vi "LimelightSeekerBasic.vi"() -> ()   [LabVIEW 2018]
uses:
  <vilib>/Rock Robotics/Network Tables/NT Read Number.vi
panel:
  in  "RotError":dbl
  in  "FinalForwardMS":u32
  out "Ts":dbl
  out "PrevFOV":bool
  out "Ta":dbl
  out "error out":errorcluster
  out "RightOut":dbl
  out "LeftOut":dbl
  in  "BaseSpeed":dbl=0.3
  out "Distance":dbl
  out "Deadband":bool
  out "RightFOV":bool
  out "LeftFOV":bool
  in  "AimMin":dbl
  in  "Camera angle":dbl=14.5
  in  "Camera height":dbl=0.3
  in  "Target height":dbl=1.4
  in  "kPDrive":dbl=1.0
  in  "kPAim":dbl=0.01
  in  "Translation Deadband":dbl=1.2
  in  "Target Area":dbl=16.0
  # "<-- This guy is a percentage of the image in decimal format. He can't go over 1.0 or below 0.0"
  # "<-- This guy is the \"acceptable\" translational error"
  # "<-- Proportionality constants"
  # "<-- Height of your target. This VARIES w cargo ship and rocket so we need a selector (thats a TODO)"
  # "<-- Height of camera from the ground"
  # "<-- Angle Camera makes from horizontal"
  # "<-- Minimum speed to adjust steering by, to avoid overshoot"
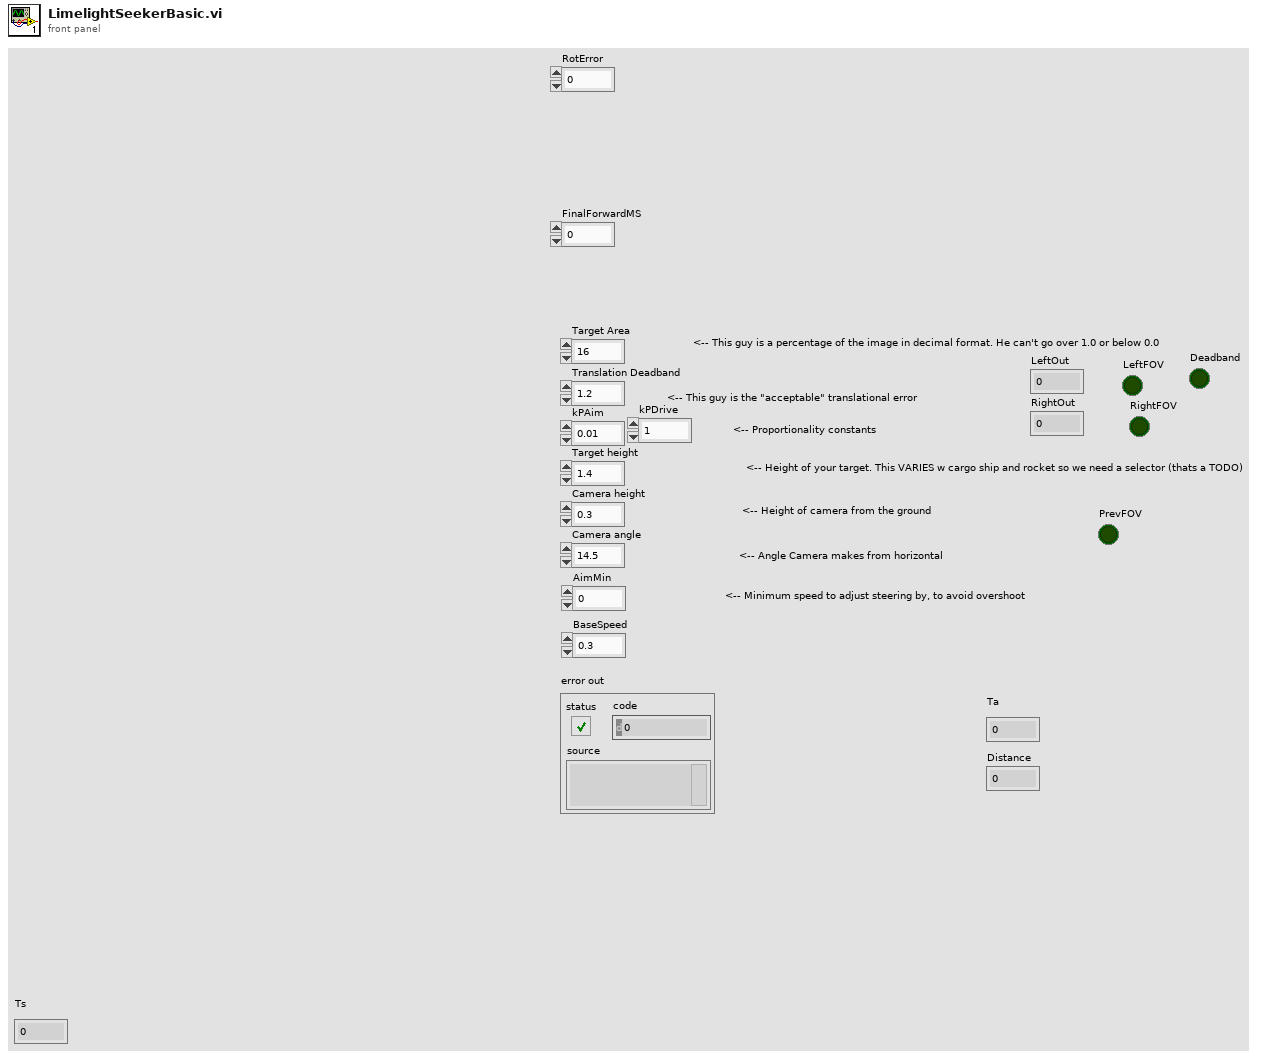
[diagram p1: front panel]
types:
  T1 = typedef "WPI_MotorControlDeviceRef.ctl" = cluster{"DeviceStatus":errorcluster, "Type":T2, "PWM":cluster{"PWM Channel":T3, "DeadBand":T4}, "CAN":cluster{"Device Number":u8, "SetOutput VI Ref":variant, "GetOutput VI Ref":variant, "Enable VI Ref":variant, "Disable VI Ref":variant, "Data":variant}, "Invert":bool, "DIO PWM":cluster{"PWM \"Enable\" Channel":T3, "DIOChannel":T5, "PWM Rate":dbl}}
  T2 = typedef "WPI_MotorControlType.ctl" = enum16{"PWM", "CAN", "DIO PWM"}
  T3 = typedef "FPGA_DIOPWMChannel.ctl" = enum8{"PWM 0", "PWM 1", "PWM 2", "PWM 3", "PWM 4", "PWM 5", "PWM 6", "PWM 7", "PWM 8", "PWM 9", "PWM MXP 0", "PWM MXP 1", "PWM MXP 2", "PWM MXP 3", "PWM MXP 4", "PWM MXP 5", "PWM MXP 6", "PWM MXP 7", "PWM MXP 8", "PWM MXP 9", "Invalid"}
  T4 = typedef "WPI_PWMDeadband.ctl" = cluster{"Name":string, "maxPositivePwm":i32, "minPositivePwm":i32, "centerPwm":i32, "maxNegativePwm":i32, "minNegativePwm":i32, "angularRange":u16}
  T5 = typedef "FPGA_DIOChannel.ctl" = enum8{"DIO 0", "DIO 1", "DIO 2", "DIO 3", "DIO 4", "DIO 5", "DIO 6", "DIO 7", "DIO 8", "DIO 9", "DIO MXP 0", "DIO MXP 1", "DIO MXP 2", "DIO MXP 3", "DIO MXP 4", "DIO MXP 5", "DIO MXP 6", "DIO MXP 7", "DIO MXP 8", "DIO MXP 9", "DIO MXP 10", "DIO MXP 11", "DIO MXP 12", "DIO MXP 13", "DIO MXP 14", "DIO MXP 15", "SPI Port CS1", "SPI Port CS2", "SPI Port CS3", "SPI Port MISO", "SPI Port MOSI", "Invalid"}
  T6 = cluster{"MotorControlDevRef":T1, "MotorControlDevRef":T1}
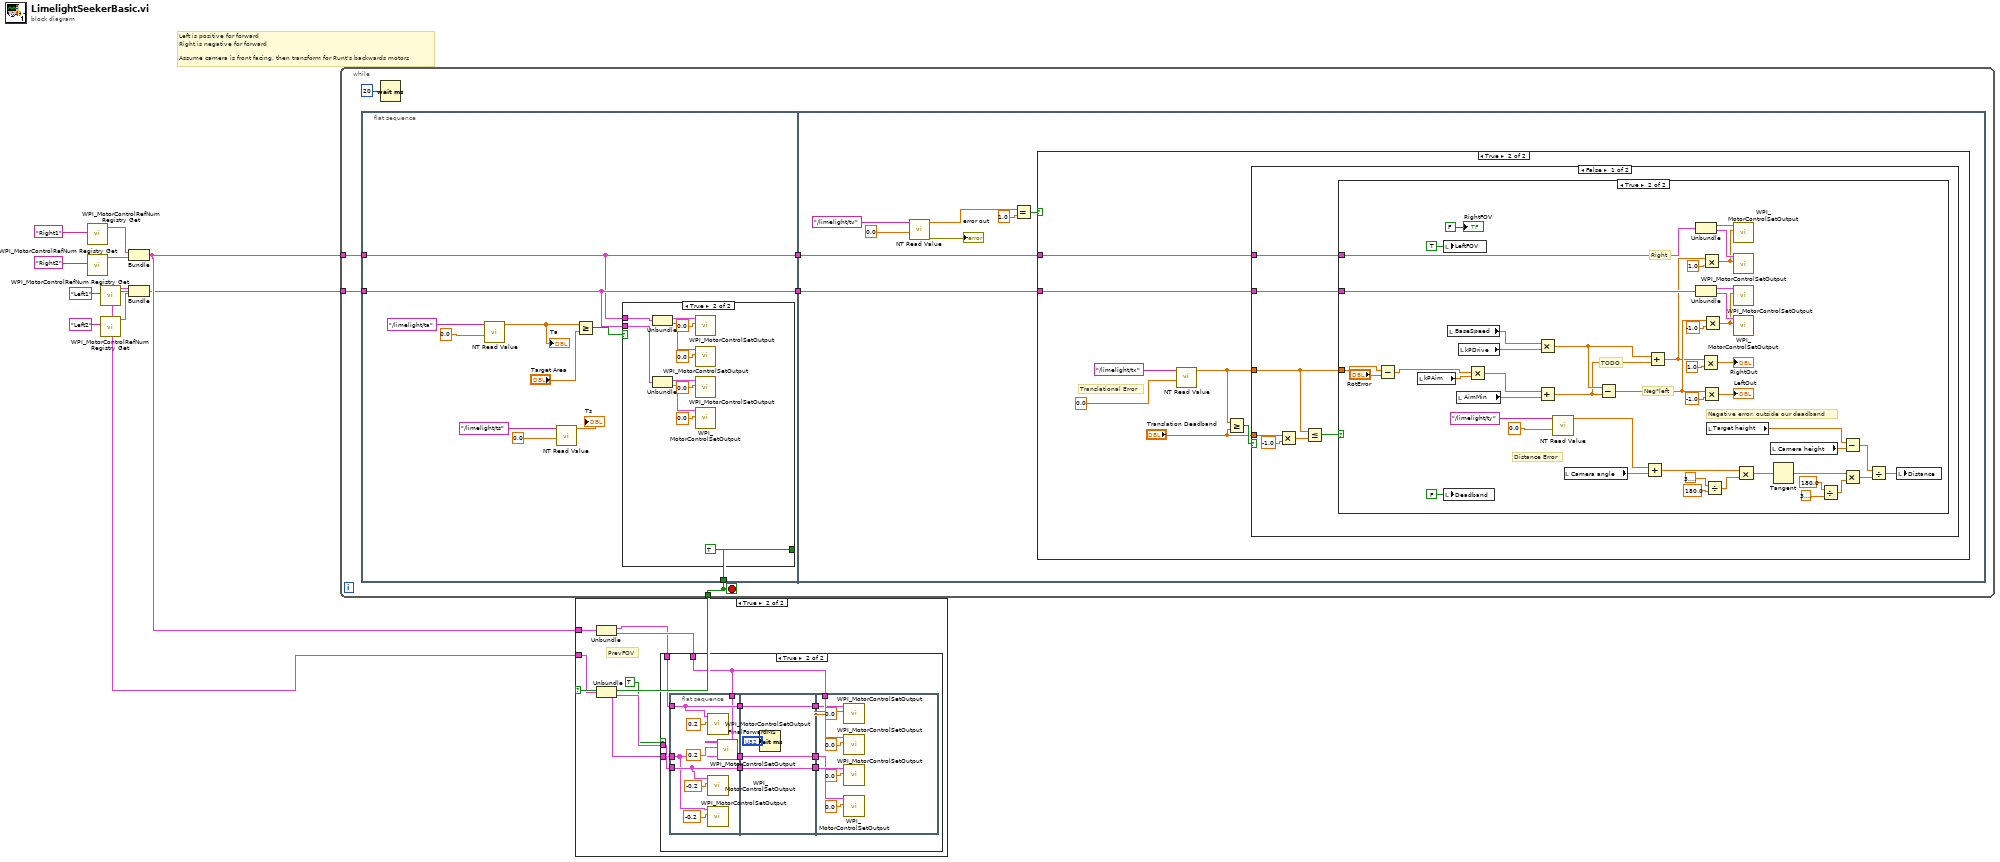
[diagram p0: block diagram]
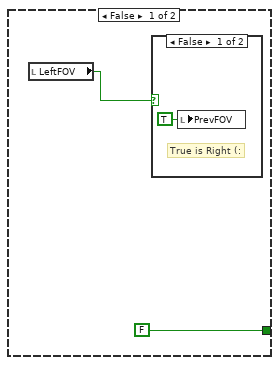
[diagram p4: hidden frame]
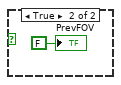
[diagram p5: hidden frame]
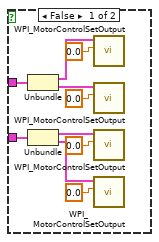
[diagram p6: hidden frame]
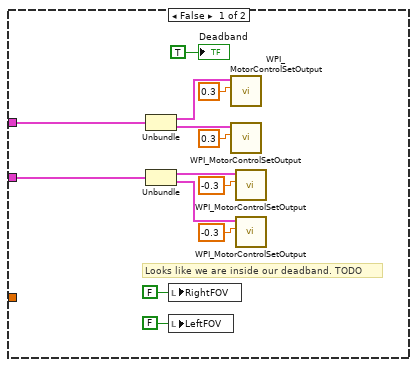
[diagram p7: hidden frame]
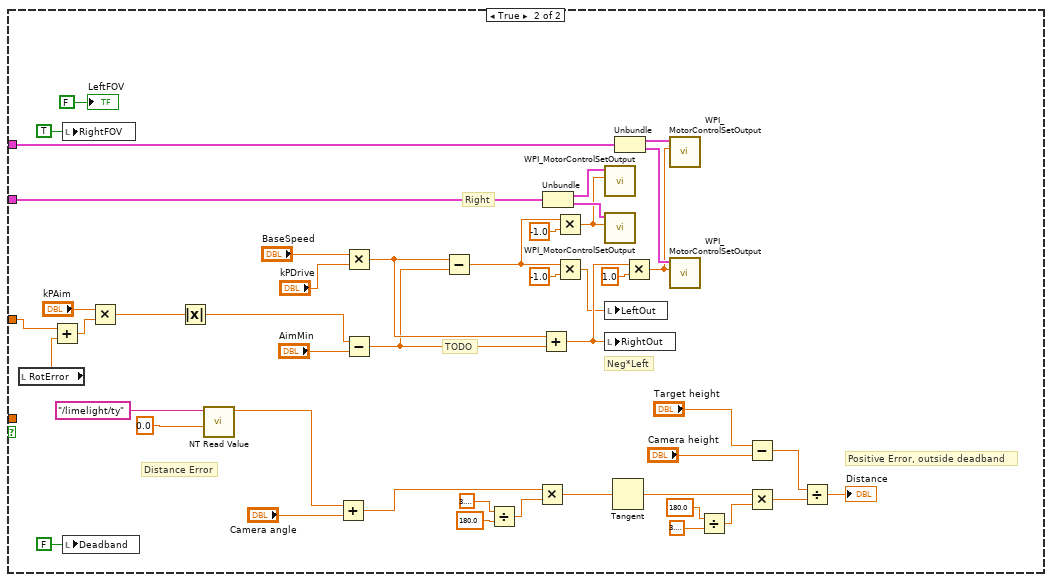
[diagram p8: hidden frame]
diagram:
  # "Left is positive for forward\nRight is negative for forward\n\nAssume camera is front facing, then transform for Runt's backwards motors"
  n1 = call <vilib>:"WPI_MotorControlRefNum Registry Get.vi"("refnum name"="Right1") -> ("MotorControlDevRef"=w5:T1)  [unwired: 9 in, 1 out]
  n2 = call <vilib>:"WPI_MotorControlRefNum Registry Get.vi"("refnum name"="Right2") -> ("MotorControlDevRef"=w4:T1)  [unwired: 9 in, 1 out]
  n3 = call <vilib>:"WPI_MotorControlRefNum Registry Get.vi"("refnum name"="Left1") -> ("MotorControlDevRef"=w7:T1)  [unwired: 9 in, 1 out]
  n4 = call <vilib>:"WPI_MotorControlRefNum Registry Get.vi"("refnum name"="Left2") -> ("MotorControlDevRef"=w6:T1)  [unwired: 9 in, 1 out]
  n5 = Bundle("MotorControlDevRef"=w5, "MotorControlDevRef"=w4) -> (w2:T6)  [unwired: 1 in]
  n6 = Bundle("MotorControlDevRef"=w7, "MotorControlDevRef"=w6) -> (w1:T6)  [unwired: 1 in]
  n7 = while {
    tunnel: w1 -> [w17]
    tunnel: w2 -> [w16]
    tunnel: [w12] -> w3
    stop <- w12 stop-if-true
    n8 = flat-sequence {
      tunnel: w16 -> [w24]
      tunnel: w17 -> [w25]
      tunnel: [w25] -> w15
      tunnel: [w24] -> w14
      tunnel: [w21] -> w12
      tunnel: w15 -> [w51]
      tunnel: w14 -> [w50]
      frame #0 {
        n9 = call-poly <vilib>:"NT Read Value.vi"("Default Value"=0.0, "Name"="/limelight/ta") -> ("Numeric"=w26:dbl)  [unwired: 8 in, 1 out]
        "Ta" <- w26
        n10 = call-poly <vilib>:"NT Read Value.vi"("Default Value"=0.0, "Name"="/limelight/ts") -> ("Numeric"=→"Ts":dbl)  [unwired: 8 in, 1 out]
        n11 = Greater Or Equal?(x=w26, y="Target Area") -> (x >= y?=w28:bool)
        n12 = case shown="True" w28 {
          tunnel: w25 -> [_ w43]
          tunnel: w24 -> [_ w42]
          tunnel: [FALSE TRUE] -> w21
          frame False {
            n13 = local read "LeftFOV"() -> (w29:bool)
            n14 = case shown="False" w29 {
              frame False {
                # "True is Right (:"
                n15 = local write "PrevFOV"(TRUE ("PrevFOV")) -> ()
              }
              frame True {
                "PrevFOV" <- FALSE ("PrevFOV")
              }
            }
          }
          frame True {
            n16 = Unbundle(w42) -> ("MotorControlDevRef"=w37:T1, "MotorControlDevRef"=w36:T1)
            n17 = Unbundle(w43) -> ("MotorControlDevRef"=w35:T1, "MotorControlDevRef"=w34:T1)
            n18 = call <vilib>:"WPI_MotorControlSetOutput.vi"("Output"=0.0, "MotorControlDevRef"=w37) -> ()  [unwired: 7 in, 3 out]
            n19 = call <vilib>:"WPI_MotorControlSetOutput.vi"("Output"=0.0, "MotorControlDevRef"=w36) -> ()  [unwired: 7 in, 3 out]
            n20 = call <vilib>:"WPI_MotorControlSetOutput.vi"("Output"=0.0, "MotorControlDevRef"=w35) -> ()  [unwired: 7 in, 3 out]
            n21 = call <vilib>:"WPI_MotorControlSetOutput.vi"("Output"=0.0, "MotorControlDevRef"=w34) -> ()  [unwired: 7 in, 3 out]
          }
        }
      }
      frame #1 {
        n22 = call-poly <vilib>:"NT Read Value.vi"("Default Value"=0.0, "Name"="/limelight/tv") -> ("error out"=→"error out":errorcluster, "Numeric"=w47:dbl)  [unwired: 8 in]
        n23 = Equal?(x=w47, y=1.0) -> (x = y?=w48:bool)
        n24 = case shown="True" w48 {
          tunnel: w51 -> [w52 w63]
          tunnel: w50 -> [w53 w62]
          frame False {
            n25 = Unbundle(w53) -> ("MotorControlDevRef"=w55:T1, "MotorControlDevRef"=w54:T1)
            n26 = Unbundle(w52) -> ("MotorControlDevRef"=w57:T1, "MotorControlDevRef"=w56:T1)
            n27 = call <vilib>:"WPI_MotorControlSetOutput.vi"("Output"=0.0, "MotorControlDevRef"=w55) -> ()  [unwired: 7 in, 3 out]
            n28 = call <vilib>:"WPI_MotorControlSetOutput.vi"("Output"=0.0, "MotorControlDevRef"=w54) -> ()  [unwired: 7 in, 3 out]
            n29 = call <vilib>:"WPI_MotorControlSetOutput.vi"("Output"=0.0, "MotorControlDevRef"=w57) -> ()  [unwired: 7 in, 3 out]
            n30 = call <vilib>:"WPI_MotorControlSetOutput.vi"("Output"=0.0, "MotorControlDevRef"=w56) -> ()  [unwired: 7 in, 3 out]
          }
          frame True {
            # "Translational Error"
            n31 = call-poly <vilib>:"NT Read Value.vi"("Default Value"=0.0, "Name"="/limelight/tx") -> ("Numeric"=w65:dbl)  [unwired: 8 in, 1 out]
            n32 = Greater Or Equal?(x=w65, y="Translation Deadband") -> (x >= y?=w66:bool)
            n33 = case shown="False" w66 {
              tunnel: w65 -> [w71 w137]
              tunnel: "Translation Deadband" -> [w73 _]
              tunnel: w63 -> [w70 w154]
              tunnel: w62 -> [w69 w153]
              frame False {
                n34 = Multiply(x=w73, y=-1.0) -> (x*y=w74:dbl)
                n35 = Less Or Equal?(x=w71, y=w74) -> (x <= y?=w72:bool)
                n36 = case shown="True" w72 {
                  tunnel: w71 -> [_ w90]
                  tunnel: w70 -> [w76 w107]
                  tunnel: w69 -> [w77 w106]
                  frame False {
                    # "Looks like we are inside our deadband. TODO"
                    n37 = Unbundle(w77) -> ("MotorControlDevRef"=w79:T1, "MotorControlDevRef"=w78:T1)
                    n38 = Unbundle(w76) -> ("MotorControlDevRef"=w81:T1, "MotorControlDevRef"=w80:T1)
                    n39 = local write "RightFOV"(FALSE ("RightFOV")) -> ()
                    n40 = local write "LeftFOV"(FALSE ("LeftFOV")) -> ()
                    n41 = call <vilib>:"WPI_MotorControlSetOutput.vi"("Output"=0.3, "MotorControlDevRef"=w79) -> ()  [unwired: 7 in, 3 out]
                    n42 = call <vilib>:"WPI_MotorControlSetOutput.vi"("Output"=0.3, "MotorControlDevRef"=w78) -> ()  [unwired: 7 in, 3 out]
                    n43 = call <vilib>:"WPI_MotorControlSetOutput.vi"("Output"=-0.3, "MotorControlDevRef"=w81) -> ()  [unwired: 7 in, 3 out]
                    n44 = call <vilib>:"WPI_MotorControlSetOutput.vi"("Output"=-0.3, "MotorControlDevRef"=w80) -> ()  [unwired: 7 in, 3 out]
                    "Deadband" <- TRUE ("Deadband")
                  }
                  frame True {
                    # "Right"
                    # "Neg*left"
                    # "TODO"
                    # "Distance Error"
                    # "Negative error, outside our deadband"
                    n45 = Subtract(x=w90, y="RotError") -> (x-y=w89:dbl)
                    n46 = local read "kPAim"() -> (w124:dbl)
                    n47 = local write "LeftFOV"(TRUE ("LeftFOV")) -> ()
                    n48 = local write "Deadband"(FALSE ("Deadband")) -> ()
                    n49 = local read "BaseSpeed"() -> (w109:dbl)
                    n50 = local read "AimMin"() -> (w123:dbl)
                    n51 = local read "kPDrive"() -> (w125:dbl)
                    n52 = Multiply(x=w89, y=w124) -> (x*y=w131:dbl)
                    n53 = Multiply(x=w109, y=w125) -> (x*y=w130:dbl)
                    n54 = Add(x=w131, y=w123) -> (x+y=w129:dbl)
                    n55 = call-poly <vilib>:"NT Read Value.vi"("Default Value"=0.0, "Name"="/limelight/ty") -> ("Numeric"=w133:dbl)  [unwired: 8 in, 1 out]
                    n56 = local read "Camera angle"() -> (w126:dbl)
                    n57 = Subtract(x=w130, y=w129) -> (x-y=w97:dbl)
                    n58 = Add(x=w133, y=w126) -> (x+y=w111:dbl)
                    n59 = Add(x=w130, y=w129) -> (x+y=w93:dbl)
                    n60 = Unbundle(w106) -> ("MotorControlDevRef"=w102:T1, "MotorControlDevRef"=w101:T1)
                    n61 = Unbundle(w107) -> ("MotorControlDevRef"=w104:T1, "MotorControlDevRef"=w103:T1)
                    n62 = Multiply(x=w93, y=1.0) -> (x*y=→"RightOut":dbl)
                    n63 = Multiply(x=w93, y=1.0) -> (x*y=w99:dbl)
                    n64 = Multiply(x=w97, y=-1.0) -> (x*y=→"LeftOut":dbl)
                    n65 = Multiply(x=w97, y=-1.0) -> (x*y=w100:dbl)
                    n66 = Divide(x=3.141592653589793, y=180.0) -> (x/y=w119:dbl)
                    n67 = local read "Target height"() -> (w128:dbl)
                    n68 = call <vilib>:"WPI_MotorControlSetOutput.vi"("Output"=w99, "MotorControlDevRef"=w102) -> ()  [unwired: 7 in, 3 out]
                    n69 = call <vilib>:"WPI_MotorControlSetOutput.vi"("Output"=w99, "MotorControlDevRef"=w101) -> ()  [unwired: 7 in, 3 out]
                    n70 = call <vilib>:"WPI_MotorControlSetOutput.vi"("Output"=w100, "MotorControlDevRef"=w104) -> ()  [unwired: 7 in, 3 out]
                    n71 = call <vilib>:"WPI_MotorControlSetOutput.vi"("Output"=w100, "MotorControlDevRef"=w103) -> ()  [unwired: 7 in, 3 out]
                    n72 = Multiply(x=w111, y=w119) -> (x*y=w108:dbl)
                    n73 = local read "Camera height"() -> (w127:dbl)
                    n74 = Tangent(1:w108) -> (0:w113:dbl)
                    n75 = Divide(x=180.0 ("y"), y=3.141592653589793) -> (x/y=w116:dbl)
                    n76 = Subtract(x=w128, y=w127) -> (x-y=w132:dbl)
                    n77 = Multiply(x=w113, y=w116) -> (x*y=w112:dbl)
                    n78 = Divide(x=w132, y=w112) -> (x/y=w110:dbl)
                    n79 = local write "Distance"(w110) -> ()
                    "RightFOV" <- FALSE ("RightFOV")
                  }
                }
              }
              frame True {
                # "Neg*Left"
                # "Right"
                # "TODO"
                # "Distance Error"
                # "Positive Error, outside deadband"
                n80 = local read "RotError"() -> (w136:dbl)
                n81 = Add(x=w137, y=w136) -> (x+y=w138:dbl)
                n82 = local write "RightFOV"(TRUE ("RightFOV")) -> ()
                n83 = local write "Deadband"(FALSE ("Deadband")) -> ()
                n84 = Multiply(x="kPAim", y=w138) -> (x*y=w143:dbl)
                n85 = Absolute Value(x=w143) -> (abs(x)=w142:dbl)
                n86 = call-poly <vilib>:"NT Read Value.vi"("Default Value"=0.0, "Name"="/limelight/ty") -> ("Numeric"=w175:dbl)  [unwired: 8 in, 1 out]
                n87 = Add(x=w175, y="Camera angle") -> (x+y=w160:dbl)
                n88 = Multiply(x="BaseSpeed", y="kPDrive") -> (x*y=w170:dbl)
                n89 = Subtract(x=w142, y="AimMin") -> (x-y=w169:dbl)
                n90 = Subtract(x=w170, y=w169) -> (x-y=w141:dbl)
                n91 = Divide(x=3.141592653589793, y=180.0) -> (x/y=w165:dbl)
                n92 = Multiply(x=w160, y=w165) -> (x*y=w158:dbl)
                n93 = Add(x=w170, y=w169) -> (x+y=w144:dbl)
                n94 = Unbundle(w154) -> ("MotorControlDevRef"=w151:T1, "MotorControlDevRef"=w150:T1)
                n95 = Multiply(x=w141, y=-1.0) -> (x*y=w147:dbl)
                n96 = Multiply(x=w141, y=-1.0) -> (x*y=w139:dbl)
                n97 = call <vilib>:"WPI_MotorControlSetOutput.vi"("Output"=w147, "MotorControlDevRef"=w151) -> ()  [unwired: 7 in, 3 out]
                n98 = call <vilib>:"WPI_MotorControlSetOutput.vi"("Output"=w147, "MotorControlDevRef"=w150) -> ()  [unwired: 7 in, 3 out]
                n99 = local write "LeftOut"(w139) -> ()
                n100 = local write "RightOut"(w144) -> ()
                n101 = Tangent(1:w158) -> (0:w157:dbl)
                n102 = Unbundle(w153) -> ("MotorControlDevRef"=w152:T1, "MotorControlDevRef"=w149:T1)
                n103 = Multiply(x=w144, y=1.0) -> (x*y=w145:dbl)
                n104 = call <vilib>:"WPI_MotorControlSetOutput.vi"("Output"=w145, "MotorControlDevRef"=w152) -> ()  [unwired: 7 in, 3 out]
                n105 = call <vilib>:"WPI_MotorControlSetOutput.vi"("Output"=w145, "MotorControlDevRef"=w149) -> ()  [unwired: 7 in, 3 out]
                n106 = Divide(x=180.0 ("y"), y=3.141592653589793) -> (x/y=w163:dbl)
                n107 = Subtract(x="Target height", y="Camera height") -> (x-y=w173:dbl)
                n108 = Multiply(x=w157, y=w163) -> (x*y=w156:dbl)
                n109 = Divide(x=w173, y=w156) -> (x/y=→"Distance":dbl)
                "LeftFOV" <- FALSE ("LeftFOV")
              }
            }
          }
        }
      }
    }
    n110 = Wait (ms)(milliseconds to wait=u32 20) -> ()  [unwired: 1 out]
  }
  n111 = case shown="True" w3 {
    tunnel: w2 -> [_ w185]
    tunnel: w1 -> [_ w184]
    frame False {
    }
    frame True {
      # "PrevFOV"
      n112 = Unbundle(w185) -> ("MotorControlDevRef"=w183:T1, "MotorControlDevRef"=w188:T1)
      n113 = Unbundle(w184) -> ("MotorControlDevRef"=w187:T1, "MotorControlDevRef"=w186:T1)
      n114 = case shown="True" TRUE {
        tunnel: w188 -> [_ w195]
        tunnel: w187 -> [_ w198]
        tunnel: w186 -> [_ w197]
        tunnel: w183 -> [_ w196]
        frame False {
        }
        frame True {
          n115 = flat-sequence {
            tunnel: w196 -> [w203]
            tunnel: w197 -> [w199]
            tunnel: w198 -> [w200]
            tunnel: [w200] -> w194
            tunnel: [w199] -> w192
            tunnel: [w203] -> w190
            tunnel: w195 -> [w201]
            tunnel: w194 -> [w210]
            tunnel: [w210] -> w193
            tunnel: w192 -> [w209]
            tunnel: [w209] -> w191
            tunnel: w190 -> [w208]
            tunnel: [w208] -> w189
            tunnel: w195 -> [w214]
            tunnel: w193 -> [w213]
            tunnel: w191 -> [w212]
            tunnel: w189 -> [w211]
            frame #0 {
              n116 = call <vilib>:"WPI_MotorControlSetOutput.vi"("Output"=0.2, "MotorControlDevRef"=w203) -> ()  [unwired: 7 in, 3 out]
              n117 = call <vilib>:"WPI_MotorControlSetOutput.vi"("Output"=-0.2, "MotorControlDevRef"=w200) -> ()  [unwired: 7 in, 3 out]
              n118 = call <vilib>:"WPI_MotorControlSetOutput.vi"("Output"=-0.2, "MotorControlDevRef"=w199) -> ()  [unwired: 7 in, 3 out]
              n119 = call <vilib>:"WPI_MotorControlSetOutput.vi"("Output"=0.2, "MotorControlDevRef"=w201) -> ()  [unwired: 7 in, 3 out]
            }
            frame #1 {
              n120 = Wait (ms)(milliseconds to wait="FinalForwardMS") -> ()  [unwired: 1 out]
            }
            frame #2 {
              n121 = call <vilib>:"WPI_MotorControlSetOutput.vi"("Output"=0.0, "MotorControlDevRef"=w211) -> ()  [unwired: 7 in, 3 out]
              n122 = call <vilib>:"WPI_MotorControlSetOutput.vi"("Output"=0.0, "MotorControlDevRef"=w214) -> ()  [unwired: 7 in, 3 out]
              n123 = call <vilib>:"WPI_MotorControlSetOutput.vi"("Output"=0.0, "MotorControlDevRef"=w213) -> ()  [unwired: 7 in, 3 out]
              n124 = call <vilib>:"WPI_MotorControlSetOutput.vi"("Output"=0.0, "MotorControlDevRef"=w212) -> ()  [unwired: 7 in, 3 out]
            }
          }
        }
      }
    }
  }
